vi "AddHandler.vi"(8 "error in (no error)":errorcluster, 10 "Handler in":refnum<class "Handler.lvclass">, 11 "Logger in":refnum<class "Logger.lvclass">) -> (0 "error out":errorcluster, 2 "Handler out":refnum<class "Handler.lvclass">, 3 "Logger out":refnum<class "Logger.lvclass">)   [LabVIEW 2022 SP3, in "Logger.lvlib" / "Logger.lvclass"]
uses:
  Logger.lvclass
  Logger.lvclass/Logger.ctl
  Handler/Handler.lvclass
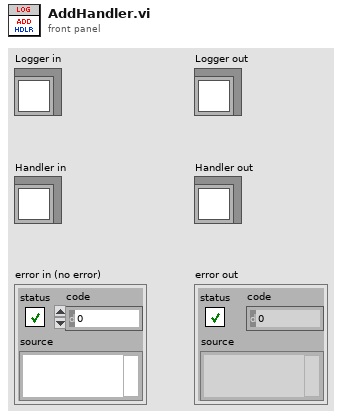
[diagram p1: front panel]
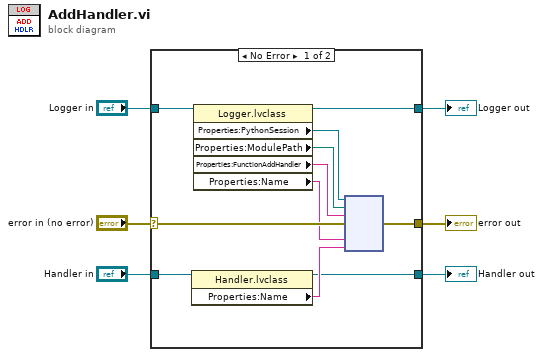
[diagram p0: block diagram]
diagram:
  n1 = case shown="No Error" "error in (no error)" {
    selector: "error in (no error)" -> [w15 w19]
    tunnel: [w14 w19] -> w3
    tunnel: [w16 w18] -> w5
    tunnel: "Logger in" -> [w17 w18]
    tunnel: "Handler in" -> [w9 _]
    tunnel: [w7 _] -> w1
    frame No Error {
      n2 = property class="Handler.lvclass"(reference=w9) -> (reference out=w7:refnum<class "Handler.lvclass">, "Properties:Name"=w8:string)  [unwired: 1 in, 1 out]
      n3 = property class="Logger.lvclass"(reference=w17) -> (reference out=w16:refnum<class "Logger.lvclass">, "Properties:PythonSession"=w13:refnum<k35>, "Properties:ModulePath"=w11:path, "Properties:FunctionAddHandler"=w12:string, "Properties:Name"=w10:string)  [unwired: 1 in, 1 out]
      n4 = node(w13, w11, w12, w15, w10, w8) -> (w14:errorcluster)  [unwired: 4 in, 3 out]
    }
    frame Error {
    }
  }
  "error out" <- w3
  "Logger out" <- w5
  "Handler out" <- w1
